vi "Init - No allocation.vi"(5 "I/O timing (ns)":T1, 8 "error in (no error)":errorcluster, 9 "Default transition action":T2, 10 "Sample rate":dbl format="%#_6p", 11 "I2C timing (ns)":T3 {"fSCL" format="%#_6p"}) -> (0 "error out":errorcluster, 1 "Coerced I/O timing (ns)":T1, 2 "Coerced I2C timing (ns)":T3 {"fSCL" format="%#_6p"}, 3 "I2C waveform info":T4)   [LabVIEW 2009, in "IDW.lvlib"]
doc: "Initializes an I2C waveform. Timing parameters are coerced to edges at the given sample rate. The coerced values are output from the VI.\n\nThis is a polymorphic instance of the <b>Init</b> VI. In this instance, buffers are preallocated in memory for the I2C waveform generation operations."
uses:
  IDW.lvlib
  _Typedefs/Waveform info.ctl
  _Typedefs/Timing - ticks.ctl
  _Typedefs/Default transition action.ctl
  _Typedefs/Bit type.ctl
  _Typedefs/Timing - ns.ctl
  _Typedefs/IO timing - ns.ctl
panel:
  # "30-70% rise requested instead of 0-30% so scope measurement is more accurate."
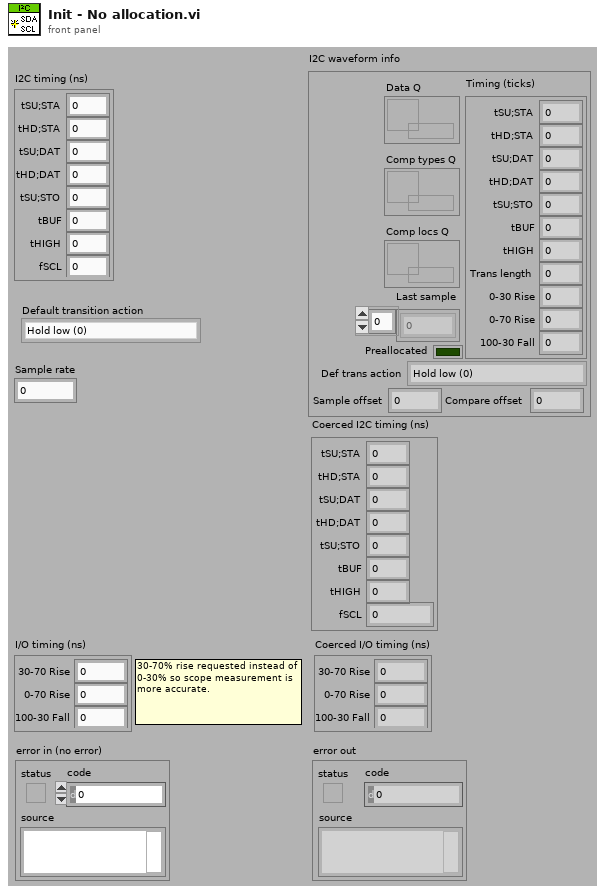
[diagram p1: front panel]
types:
  T1 = typedef "IDW.lvlib/IO timing - ns.ctl" = cluster{"30-70 Rise":dbl, "0-70 Rise":dbl, "100-30 Fall":dbl}
  T2 = typedef "IDW.lvlib/Default transition action.ctl" = enum16{"Hold low (0)", "Release (Z)", "Set up next value", "Hold previous value", "Preserve tHD;DAT and tSU;DAT"}
  T3 = typedef "IDW.lvlib/Timing - ns.ctl" = cluster{"tSU;STA":i32, "tHD;STA":i32, "tSU;DAT":i32, "tHD;DAT":i32, "tSU;STO":i32, "tBUF":i32, "tHIGH":i32, "fSCL":dbl}
  T4 = typedef "IDW.lvlib/Waveform info.ctl" = cluster{"Last sample":u8[], "Sample offset":u64, "Compare offset":u64, "Timing (ticks)":T5, "Preallocated":bool, "Def trans action":T2, "Data Q":refnum<queue>, "Comp types Q":refnum<queue>, "Comp locs Q":refnum<queue>}
  T5 = typedef "IDW.lvlib/Timing - ticks.ctl" = cluster{"tSU;STA":i32, "tHD;STA":i32, "tSU;DAT":i32, "tHD;DAT":i32, "tSU;STO":i32, "tBUF":i32, "tHIGH":i32, "Trans length":i32, "0-30 Rise":i32, "0-70 Rise":i32, "100-30 Fall":i32}
  T6 = typedef "IDW.lvlib/Bit type.ctl" = enum16{"ACK", "Data"}
  T7 = cluster{"tSU;STA":dbl, "tHD;STA":dbl, "tSU;DAT":dbl, "tHD;DAT":dbl, "tSU;STO":dbl, "tBUF":dbl, "tHIGH":dbl, "fSCL":dbl}
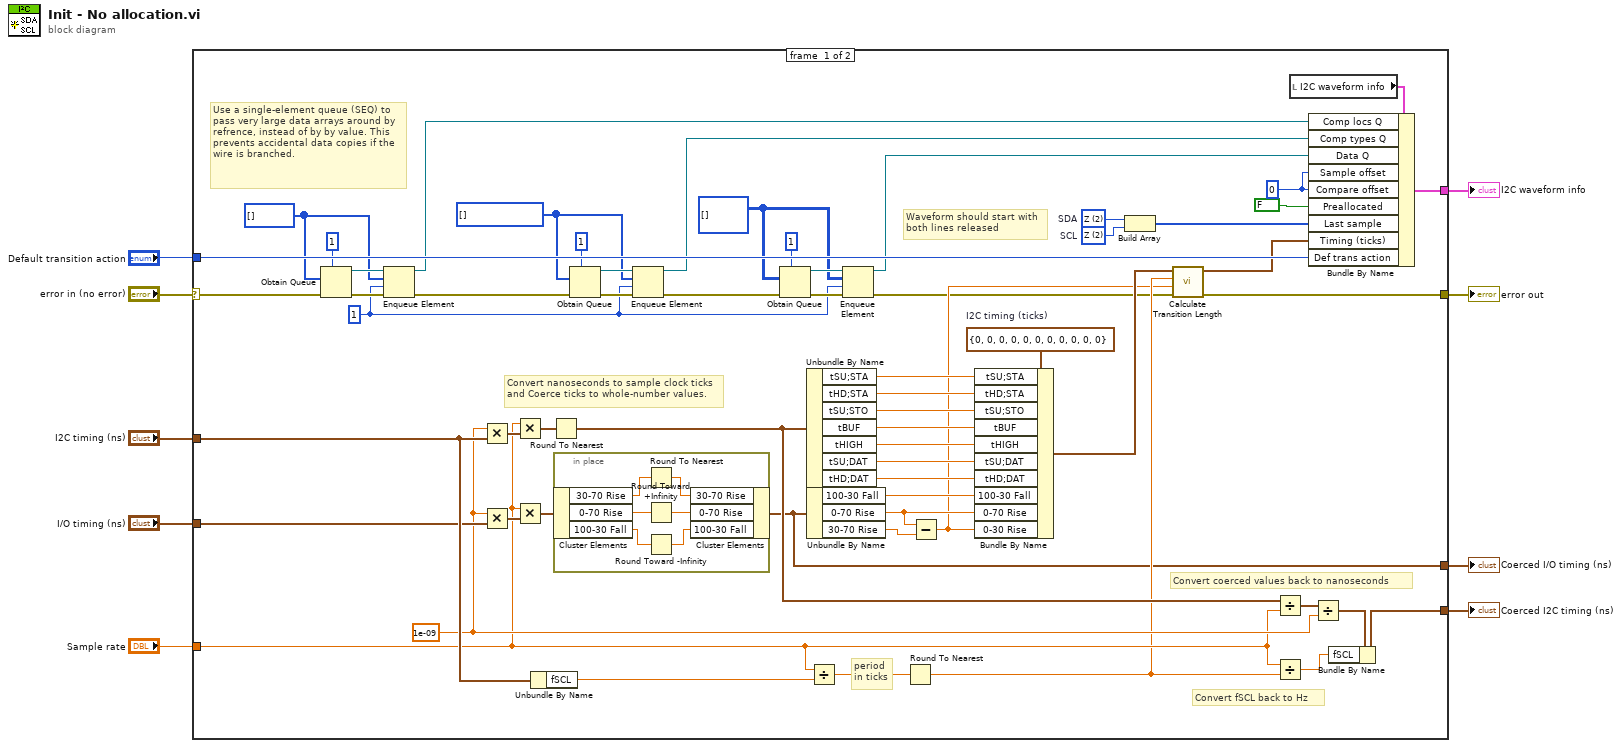
[diagram p0: block diagram]
diagram:
  n1 = case shown="No Error" "error in (no error)" {
    selector: "error in (no error)" -> [w20 w78]
    tunnel: [w67 _] -> w6
    tunnel: "I2C timing (ns)" -> [w53 w77]
    tunnel: "Sample rate" -> [w39 _]
    tunnel: [w38 w78] -> w7
    tunnel: [w55 w77] -> w4
    tunnel: "I/O timing (ns)" -> [w49 w76]
    tunnel: "Default transition action" -> [w51 _]
    tunnel: [w32 w76] -> w1
    frame #0 {
      w10 = 1 ("timeout in ms (-1)")
      w16 = u8[][] [] ("initialized array")
      w18 = T6[] [] items=["ACK", "Data"] ("initialized array")
      w17 = u64[] [] ("initialized array")
      w15 = u64 0 ("Offset")
      w41 = T5 {"tSU;STA"=0, "tHD;STA"=0, "tSU;DAT"=0, "tHD;DAT"=0, "tSU;STO"=0, "tBUF"=0, "tHIGH"=0, "Trans length"=0, "0-30 Rise"=0, "0-70 Rise"=0, "100-30 Fall"=0}  # I2C timing (ticks)
      w48 = 1e-09
      w69 = u8 2 items=["0", "1", "Z", "L", "H", "X", "T", "V"]  # SCL
      w68 = u8 2 items=["0", "1", "Z", "L", "H", "X", "T", "V"]  # SDA
      # "Use a single-element queue (SEQ) to pass very large data arrays around by refrence, instead of by by value. This prevents accidental data copies if the wire is branched."
      # "Convert fSCL back to Hz"
      # "period\nin ticks"
      # "Waveform should start with  both lines released"
      # "Convert coerced values back to nanoseconds"
      # "Convert nanoseconds to sample clock ticks and Coerce ticks to whole-number values."
      n2 = Obtain Queue(max queue size (-1, unlimited)=1, element data type=w17, error in (no error)=w20) -> (queue out=w30:refnum<queue>, error out=w31:errorcluster)  [unwired: 2 in, 1 out]
      n3 = Enqueue Element(queue=w30, element=w17, timeout in ms (-1)=w10, error in (no error)=w31) -> (queue out=w11:refnum<queue>, error out=w25:errorcluster)  [unwired: 1 out]
      n4 = Multiply(x=w48, y=w53) -> (x*y=w64:T7)
      n5 = Multiply(x=w48, y=w49) -> (x*y=w50:T1)
      n6 = Multiply(x=w39, y=w64) -> (x*y=w54:T7)
      n7 = Multiply(x=w39, y=w50) -> (x*y=w33:T1)
      n8 = Unbundle By Name(w53) -> ("fSCL"=w58:dbl)
      n9 = Round To Nearest(number=w54) -> (nearest integer value=w40:T7)
      n10 = in-place {
        n11 = in-place-cluster #1(w33) -> ("30-70 Rise"=w71:dbl, "0-70 Rise"=w73:dbl, "100-30 Fall"=w75:dbl)
        n12 = Round To Nearest(number=w71) -> (nearest integer value=w70:dbl)
        n13 = Round Toward +Infinity(x=w73) -> (ceil(x): smallest int >= x=w72:dbl)
        n14 = Round Toward -Infinity(1:w75) -> (0:w74:dbl)
        n15 = in-place-cluster #1("30-70 Rise"=w70, "0-70 Rise"=w72, "100-30 Fall"=w74) -> (w32:T1)
      }
      n16 = Obtain Queue(max queue size (-1, unlimited)=1, element data type=w18, error in (no error)=w25) -> (queue out=w27:refnum<queue>, error out=w26:errorcluster)  [unwired: 2 in, 1 out]
      n17 = Enqueue Element(queue=w27, element=w18, timeout in ms (-1)=w10, error in (no error)=w26) -> (queue out=w12:refnum<queue>, error out=w21:errorcluster)  [unwired: 1 out]
      n18 = Obtain Queue(max queue size (-1, unlimited)=1, element data type=w16, error in (no error)=w21) -> (queue out=w23:refnum<queue>, error out=w24:errorcluster)  [unwired: 2 in, 1 out]
      n19 = Unbundle By Name(w40) -> ("tSU;STA"=w59:dbl, "tHD;STA"=w60:dbl, "tSU;STO"=w61:dbl, "tBUF"=w62:dbl, "tHIGH"=w46:dbl, "tSU;DAT"=w45:dbl, "tHD;DAT"=w44:dbl)
      n20 = Unbundle By Name(w32) -> ("100-30 Fall"=w43:dbl, "0-70 Rise"=w42:dbl, "30-70 Rise"=w47:dbl)
      n21 = Divide(x=w39, y=w58) -> (x/y=w57:dbl)
      n22 = Enqueue Element(queue=w23, element=w16, timeout in ms (-1)=w10, error in (no error)=w24) -> (queue out=w13:refnum<queue>, error out=w19:errorcluster)  [unwired: 1 out]
      n23 = Round To Nearest(number=w57) -> (nearest integer value=w35:dbl)
      n24 = Subtract(x=w42, y=w47) -> (x-y=w34:dbl)
      n25 = Bundle By Name(cluster=w41, "tSU;STA"=w59, "tHD;STA"=w60, "tSU;STO"=w61, "tBUF"=w62, "tHIGH"=w46, "tSU;DAT"=w45, "tHD;DAT"=w44, "100-30 Fall"=w43, "0-70 Rise"=w42, "0-30 Rise"=w34) -> (w37:T5)
      n26 = Build Array(w68, w69) -> (w65:u8[])
      n27 = call "Calculate Transition Length.vi"("error in (no error)"=w19, "30-70 Rise"=w34, "1/ fSCL"=w35, "I2C timing (ticks)"=w37) -> ("error out"=w38:errorcluster, "I2C timing (ticks) out"=w36:T5)  [unwired: 6 in]
      n28 = Divide(x=w40, y=w39) -> (x/y=w63:T7)
      n29 = Divide(x=w39, y=w35) -> (x/y=w52:dbl)
      n30 = local read "I2C waveform info"() -> (w66:T4)
      n31 = Bundle By Name(cluster=w66, "Comp locs Q"=w11, "Comp types Q"=w12, "Data Q"=w13, "Sample offset"=w15, "Compare offset"=w15, "Preallocated"=FALSE, "Last sample"=w65, "Timing (ticks)"=w36, "Def trans action"=w51) -> (w67:T4)
      n32 = Divide(x=w63, y=w48) -> (x/y=w56:T7)
      n33 = Bundle By Name(cluster=w56, "fSCL"=w52) -> (w55:T7)
    }
    frame #1 {
    }
  }
  "error out" <- w7
  "I2C waveform info" <- w6
  "Coerced I2C timing (ns)" <- w4
  "Coerced I/O timing (ns)" <- w1
